vi "get_range_table_numeric_value.vi"(7 "Range Table ID in":string, 8 "error in":errorcluster caption="error in (no error)", 10 "String Value":string, 11 "VISA resource name":refnum<visa-resource-name>) -> (0 "error out":errorcluster, 2 "I32 output":i32, 3 "VISA resource name out":refnum<visa-resource-name>)   [LabVIEW 2020, in "Rohde&Schwarz RTx Oscilloscopes.lvlib" / "rsidr_core.lvlib"]
uses:
  rsidr_core.lvlib
  _type_Operation_Fgv_RangeTable.ctl
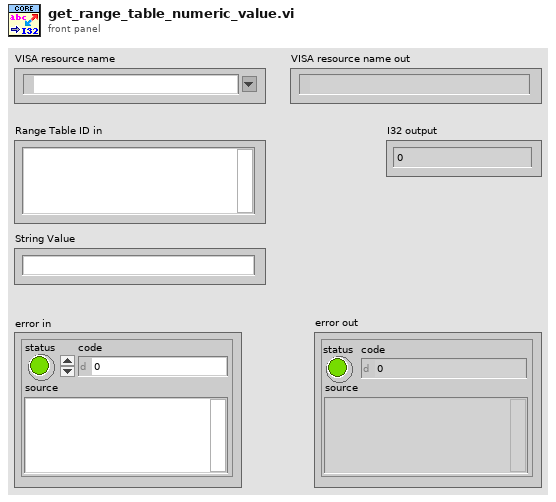
[diagram p1: front panel]
types:
  T1 = typedef "Rohde&Schwarz RTx Oscilloscopes.lvlib/rsidr_core.lvlib/_type_Operation_Fgv_RangeTable.ctl" = enum16{"Initialize", "Check", "Coerce", "Get Command String", "Get Numeric Value", "Get Default Value", "Get Range Table Type"}
  T2 = typedef "Rohde&Schwarz RTx Oscilloscopes.lvlib/rsidr_core.lvlib/_type_RangeTable_Type.ctl" = enum16{"Ranged", "Coerced", "Discrete"}
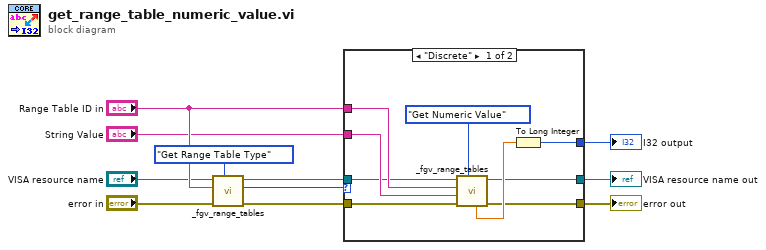
[diagram p0: block diagram]
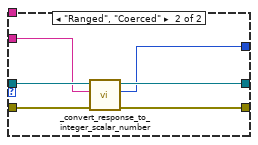
[diagram p2: hidden frame]
diagram:
  n1 = call "_fgv_range_tables.vi"("Operation"=_type_Operation_Fgv_RangeTable."Get Range Table Type", "error in"="error in", "Range Table ID in"="Range Table ID in", "VISA resource name"="VISA resource name") -> ("error out"=w5:errorcluster, "Range Table Type out"=w10:T2, "VISA resource name out"=w4:refnum<visa-resource-name>)  [unwired: 3 in, 2 out]
  n2 = case shown="\"Discrete\"" w10 {
    tunnel: "String Value" -> [w18 w22]
    tunnel: [w16 w21] -> w1
    tunnel: w5 -> [w15 w26]
    tunnel: w4 -> [w14 w25]
    tunnel: [w13 w24] -> w3
    tunnel: [w12 w23] -> w2
    tunnel: "Range Table ID in" -> [w19 _]
    frame "Discrete" {
      n3 = call "_fgv_range_tables.vi"("Operation"=_type_Operation_Fgv_RangeTable."Get Numeric Value", "error in"=w15, "String value in (\"\")"=w18, "Range Table ID in"=w19, "VISA resource name"=w14) -> ("error out"=w13:errorcluster, "VISA resource name out"=w12:refnum<visa-resource-name>, "Numeric Value out"=w17:dbl)  [unwired: 2 in, 2 out]
      n4 = To Long Integer(number=w17) -> (32bit integer=w16:i32)
    }
    frame "Ranged", "Coerced" {
      n5 = call "_convert_response_to_integer_scalar_number.vi"("error in"=w26, "Input string"=w22, "VISA resource name"=w25) -> ("error out"=w24:errorcluster, "Int32 out"=w21:i32, "VISA resource name out"=w23:refnum<visa-resource-name>)  [unwired: 6 in]
    }
  }
  "VISA resource name out" <- w2
  "error out" <- w3
  "I32 output" <- w1
